vi "Receive Panel Close Msg.vi"(8 "error in (no error)":errorcluster, 10 "PanelCloseMsg":refnum<class "PanelCloseMsg.lvclass">, 11 "MediatorBusMonitor in":refnum<class "MediatorBusMonitor.lvclass">) -> (0 "error out":errorcluster, 3 "MediatorBusMonitor out":refnum<class "MediatorBusMonitor.lvclass">)   [LabVIEW 2015, in "Mediator.lvlib" / "MediatorBusMonitor.lvclass"]
doc: "<License>\nCopyright © 2017 Composed Systems, LLC | All rights reserved\nwww.composed.io\n\nAuthor: Ethan Stern <ethan.stern@composed.io>\n\nThis software is provided \"AS IS\" WITHOUT WARRANTIES, either express or implied, AND IS FOR EDUCATIONAL PURPOSES ONLY.\n</License>"
uses:
  MediatorBusMonitor.lvclass
  AutoRegistration/ActorAutoRegistration Messages/PanelCloseMsg/PanelCloseMsg.lvclass
  MediatorBusMonitor.lvclass/MediatorBusMonitor.ctl
  <vilib>/ActorFramework/Actor/Actor.lvclass/Actor.ctl
  <vilib>/ActorFramework/Message Enqueuer/Message Enqueuer.lvclass/Message Enqueuer.ctl
  IViewable/IViewable Messages/Close Front Panel Msg/Close Front Panel Msg.lvclass/Close Front Panel Msg.ctl
  <vilib>/ActorFramework/Message Enqueuer/Init from Existing Queue.vi
  <vilib>/ActorFramework/Message Enqueuer/Enqueue.vi
  <vilib>/ActorFramework/Message Priority Queue/Priority Enqueue.vi
  <vilib>/ActorFramework/Message Enqueuer/Message Enqueuer.lvclass
  IViewable/IViewable Messages/Close Front Panel Msg/Close Front Panel Msg.lvclass
  <vilib>/ActorFramework/Actor/Actor.lvclass
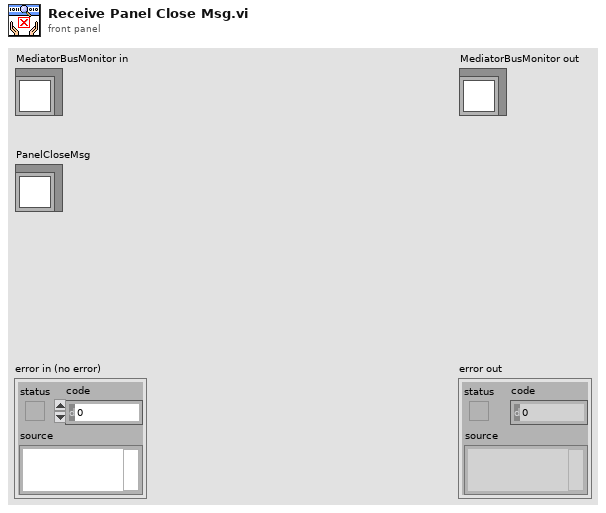
[diagram p1: front panel]
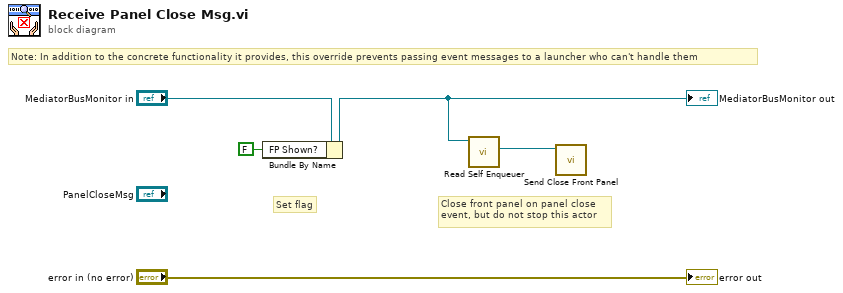
[diagram p0: block diagram]
diagram:
  # "Note: In addition to the concrete functionality it provides, this override prevents passing event messages to a launcher who can't handle them"
  # "Set flag"
  # "Close front panel on panel close\nevent, but do not stop this actor"
  n1 = Bundle By Name(cluster="MediatorBusMonitor in", "FP Shown?"=FALSE) -> (w2:refnum<class "MediatorBusMonitor.lvclass">)
  "MediatorBusMonitor out" <- w2
  n2 = call <vilib>:"Read Self Enqueuer.vi"("Actor"=w2) -> ("Self Enqueuer"=w3:refnum<class "Message Enqueuer.lvclass">)  [unwired: 10 in]
  n3 = call "Send Close Front Panel.vi"("Message Enqueuer"=w3) -> ()  [unwired: 9 in, 2 out]
  "error out" <- "error in (no error)"
